vi "Facade 1.vi"(0 "Data In":T5, 2 "Display State In":T3={"Header"="", "Label[]"=[], "DisableButtonsLUT"=variant(string[] []), "Menu Config"=variant}, 3 "Container State":T4) -> (6 "Data Out":T5, 7 "Display State Out":T3={"Header"="", "Label[]"=[], "DisableButtonsLUT"=variant(string[] []), "Menu Config"=variant}, 8 "Action":T2)   [LabVIEW 2019, in "Menu Button.xctl"]
doc: "JSMA Module Template - Top Level UI 0.2.0.4\nRob Humfeld - Jet Engineering\nCopyright (c) 2019, Jet Engineering"
uses:
  Menu Button.xctl
  Data 1.ctl
  <vilib>/_xctls/Container State.ctl
  State 1.ctl
  <vilib>/_xctls/Action.ctl
  <vilib>/_xctls/XControlSupport.lvlib
panel:
  out "Header":string
  in  "Radio Button":T1(radio)
  # "1. Drop the controls that make up the appearance\nof the XControl here.\n\n2. Resize the window to fit the controls\n\n3. If the XControl is of fixed size,  make the \n window not resizable from VI Properties->Window Appearance.\n\n4. If you want the controls to automatically size when the XControl sizes, check  \"Scale all objects on front panel when window resizes\" in File->VI Properties->Window Size page.\n\n5. Show the block diagram and handle events for the controls on this panel."
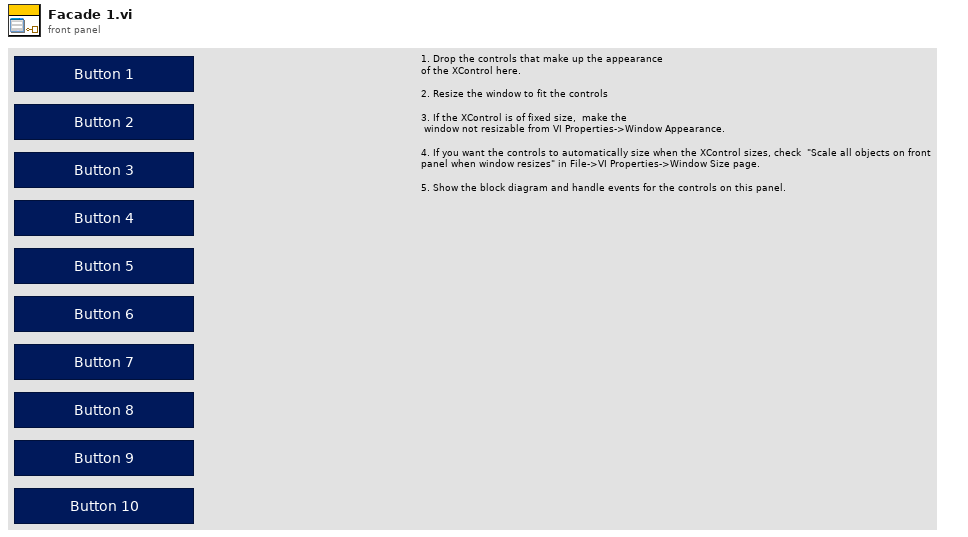
[diagram p1: front panel]
types:
  T1 = enum32{"No Selection", "System Setup", "System Monitor", "Test Selection", "Data Review", "Radio Selection 5", "Radio Selection 6", "Radio Selection 7", "Radio Selection 8", "Radio Selection 9", "Radio Selection 10"}
  T2 = typedef "XControlSupport.lvlib/Action.ctl" = cluster{"Data Changed?":bool, "State Changed?":bool, "Action Name":string}
  T3 = typedef "Menu Button.xctl/State 1.ctl" = cluster{"Header":string, "Label[]":string[], "DisableButtonsLUT":variant, "Menu Config":variant}
  T4 = typedef "XControlSupport.lvlib/Container State.ctl" = cluster{"Indicator?":bool, "Run Mode?":bool, " Refnum":refnum<vi>}
  T5 = typedef "Menu Button.xctl/Data 1.ctl" = cluster{"Button Pressed":string, "Level":string, "Menu Config":variant}
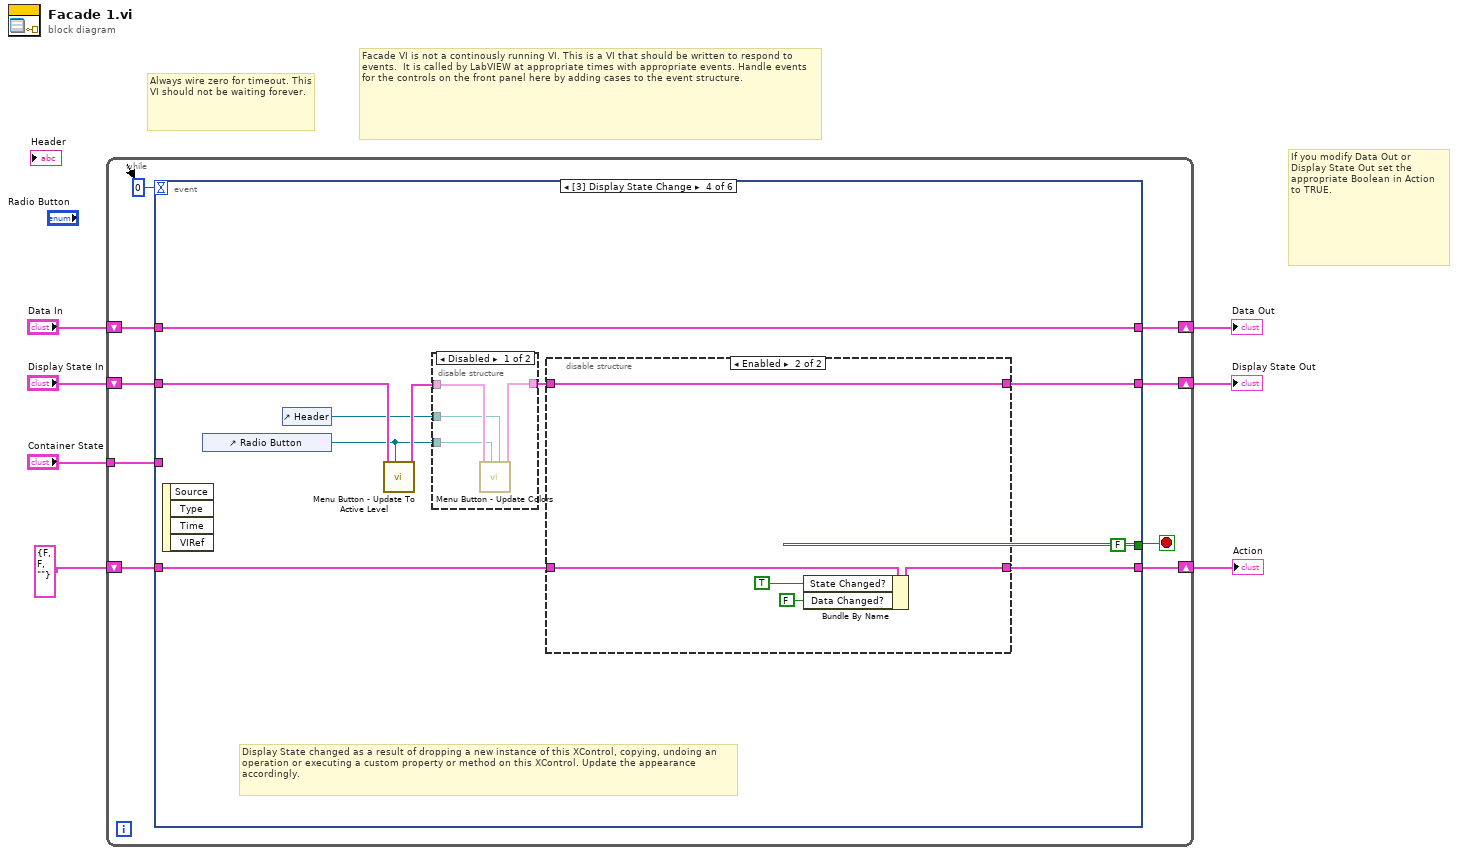
[diagram p0: block diagram]
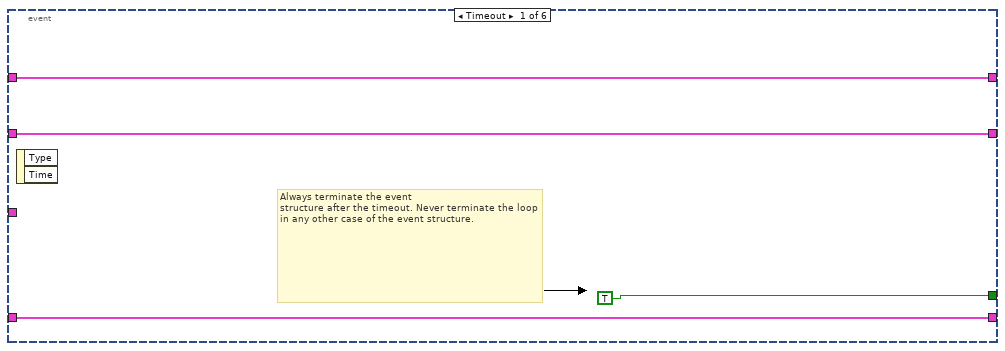
[diagram p2: hidden frame]
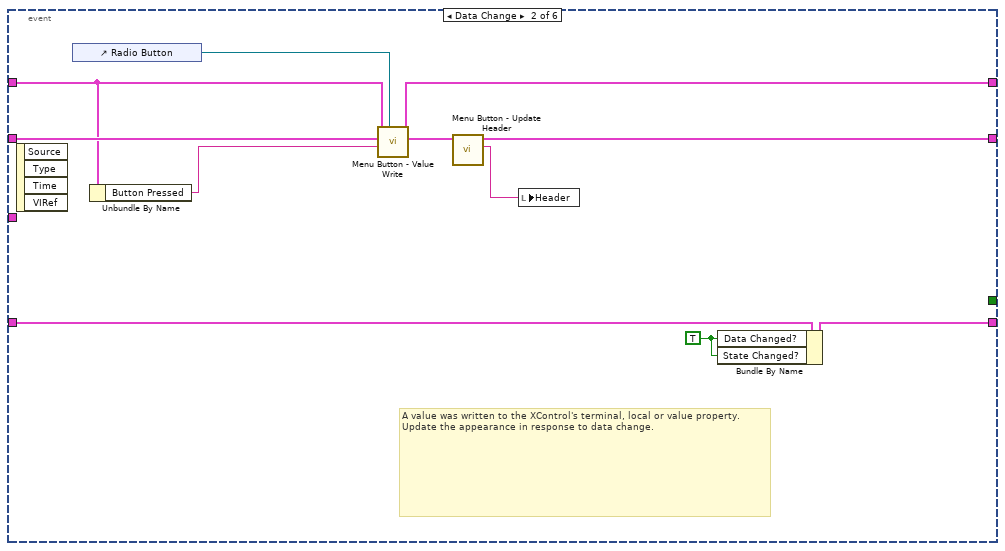
[diagram p3: hidden frame]
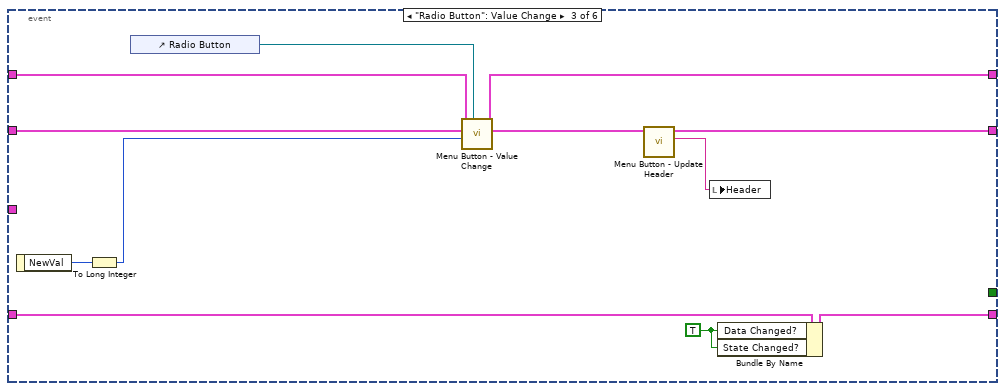
[diagram p4: hidden frame]
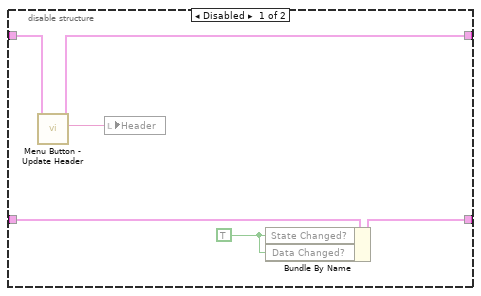
[diagram p6: hidden frame]
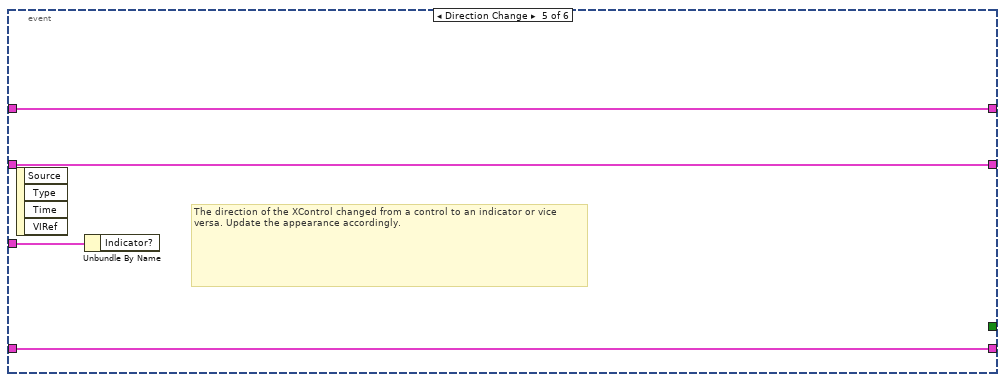
[diagram p7: hidden frame]
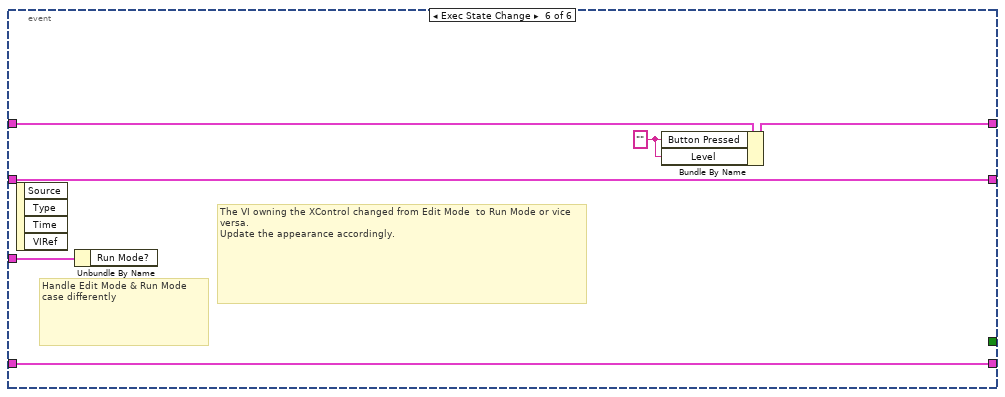
[diagram p8: hidden frame]
diagram:
  # "Facade VI is not a continously running VI. This is a VI that should be written to respond to events.  It is called by LabVIEW at appropriate times with appropriate events. Handle events for the controls on the front panel here by adding cases to the event structure."
  # "Always wire zero for timeout. This\nVI should not be waiting forever."
  # "If you modify Data Out or\nDisplay State Out set the\nappropriate Boolean in Action\nto TRUE."
  n1 = while {
    shift-right: [w15] -> w4
    shift-left: "Display State In" -> [w16]
    tunnel: "Container State" -> [w12]
    shift-right: [w10] -> w7
    shift-left: "Data In" -> [w11]
    shift-right: [w8] -> w2
    shift-left: T2 {"Data Changed?"=FALSE, "State Changed?"=FALSE, "Action Name"=""} ("Action") -> [w9]
    stop <- w14 stop-if-true
    n2 = event shown="[3] Display State Change" {
      selector: _ -> [_ _ _ _ _ _]
      dyn-events: _ -> [_ _ _ _ _ _]
      timeout: 0 -> [_ _ _ _ _ _]
      tunnel: w16 -> [w18 w30 w40 w51 w72 w78]
      tunnel: [w18 w24 w34 w48 w72 w78] -> w15
      tunnel: [TRUE _ _ FALSE _ _] -> w14
      tunnel: w12 -> [_ _ _ _ w73 w79]
      tunnel: w11 -> [w17 w29 w39 w52 w71 w77]
      tunnel: [w17 w28 w38 w52 w71 w75] -> w10
      tunnel: [w19 w22 w33 w49 w70 w76] -> w8
      tunnel: w9 -> [w19 w31 w43 w53 w70 w76]
      event Timeout {
        # "Always terminate the event\nstructure after the timeout. Never terminate the loop in any other case of the event structure."
        n3 = event-data() -> ()  [unwired: 1 in, 2 out]
      }
      event Data Change {
        w21 = TRUE ("Data Changed?")
        # "A value was written to the XControl's terminal, local or value property.\nUpdate the appearance in response to data change."
        n4 = event-data() -> ()  [unwired: 1 in, 4 out]
        n5 = control-ref of="Radio Button"() -> (w27:refnum<vi>)
        n6 = Unbundle By Name(w29) -> ("Button Pressed"=w26:string)
        n7 = call "Menu Button - Value Write.vi"("RadioButtonsControl in"=w27, "Value"=w26, "Display State In in"=w30, "Data In in"=w29) -> ("Display State In out"=w25:T3, "Data In out"=w28:T5)  [unwired: 6 in]
        n8 = call "Menu Button - Update Header.vi"("Display State In in"=w25) -> ("Header"=w23:string, "Display State In out"=w24:T3)  [unwired: 9 in]
        n9 = local write "Header"(w23) -> ()
        n10 = Bundle By Name(cluster=w31, "Data Changed?"=w21, "State Changed?"=w21) -> (w22:T2)
      }
      event "Radio Button": Value Change {
        w32 = TRUE ("Data Changed?")
        n11 = event-data() -> ("NewVal"=w42:T1)  [unwired: 1 in]
        n12 = To Long Integer(number=w42) -> (32bit integer=w41:i32)
        n13 = control-ref of="Radio Button"() -> (w37:refnum<vi>)
        n14 = call "Menu Button - Value Change.vi"("RadioButtonsControl in"=w37, "Numeric"=w41, "Display State In in"=w40, "Data In in"=w39) -> ("Display State In out"=w35:T3, "Data In out"=w38:T5)  [unwired: 6 in]
        n15 = call "Menu Button - Update Header.vi"("Display State In in"=w35) -> ("Header"=w36:string, "Display State In out"=w34:T3)  [unwired: 9 in]
        n16 = local write "Header"(w36) -> ()
        n17 = Bundle By Name(cluster=w43, "Data Changed?"=w32, "State Changed?"=w32) -> (w33:T2)
      }
      event Display State Change {
        # "Display State changed as a result of dropping a new instance of this XControl, copying, undoing an operation or executing a custom property or method on this XControl. Update the appearance accordingly."
        n18 = event-data() -> ()  [unwired: 1 in, 4 out]
        n19 = control-ref of="Radio Button"() -> (w45:refnum<vi>)
        n20 = control-ref of="Header"() -> (w44:refnum<vi>)
        n21 = call "Menu Button - Update To Active Level.vi"("RadioButtonsControl in"=w45, "Display State In in"=w51) -> ("Display State In out"=w47:T3)  [unwired: 9 in]
        n22 = disable-structure shown="Disabled" {
          disable-tunnel: w47 -> [w57 w58]
          disable-tunnel: [w56 w58] -> w46
          disable-tunnel: w45 -> [w55 _]
          disable-tunnel: w44 -> [w54 _]
          frame Disabled {
            n23 = call "Menu Button - Update Colors.vi"("Header In"=w54, "RadioButtonsControl in"=w55, "Display State In in"=w57) -> ("Display State In out"=w56:T3)  [unwired: 8 in]
          }
          frame Enabled {
          }
        }
        n24 = disable-structure shown="Enabled" {
          disable-tunnel: w53 -> [w64 w69]
          disable-tunnel: [w63 w68] -> w49
          disable-tunnel: [w61 w66] -> w48
          disable-tunnel: w46 -> [w59 w66]
          frame Disabled {
            w60 = TRUE ("State Changed?")
            n25 = call "Menu Button - Update Header.vi"("Display State In in"=w59) -> ("Header"=w62:string, "Display State In out"=w61:T3)  [unwired: 9 in]
            n26 = local write "Header"(w62) -> ()
            n27 = Bundle By Name(cluster=w64, "State Changed?"=w60, "Data Changed?"=w60) -> (w63:T2)
          }
          frame Enabled {
            n28 = Bundle By Name(cluster=w69, "State Changed?"=TRUE, "Data Changed?"=FALSE) -> (w68:T2)
          }
        }
      }
      event Direction Change {
        # "The direction of the XControl changed from a control to an indicator or vice versa. Update the appearance accordingly."
        n29 = event-data() -> ()  [unwired: 1 in, 4 out]
        n30 = Unbundle By Name(w73) -> ()  [unwired: 1 out]
      }
      event Exec State Change {
        w74 = "" ("Button Pressed")
        # "The VI owning the XControl changed from Edit Mode  to Run Mode or vice versa.\nUpdate the appearance accordingly."
        # "Handle Edit Mode & Run Mode\ncase differently"
        n31 = event-data() -> ()  [unwired: 1 in, 4 out]
        n32 = Unbundle By Name(w79) -> ()  [unwired: 1 out]
        n33 = Bundle By Name(cluster=w77, "Button Pressed"=w74, "Level"=w74) -> (w75:T5)
      }
    }
  }
  "Display State Out" <- w4
  "Data Out" <- w7
  "Action" <- w2
